vi "8164B CreateLANConnection.vi"(8 "error in":errorcluster, 11 "IP address":string="169.254.2.31") -> (0 "error out":errorcluster, 3 "KeySight 8164B control out":T1)   [LabVIEW 2018, in "KeySight 8164B LAN InstrLib.lvlib"]
uses:
  KeySight 8164B LAN InstrLib.lvlib
  typedefs/KeySight 8164B control.ctl
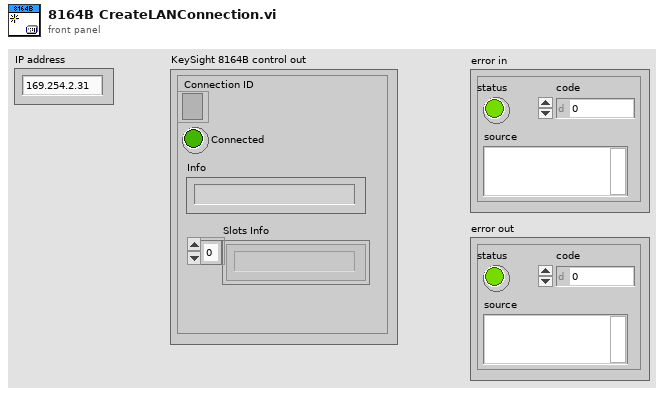
[diagram p1: front panel]
types:
  T1 = typedef "KeySight 8164B LAN InstrLib.lvlib/KeySight 8164B control.ctl" = cluster{"Connection ID":refnum<k5>, "Connected":bool, "Info":string, "Slots Info":string[]}
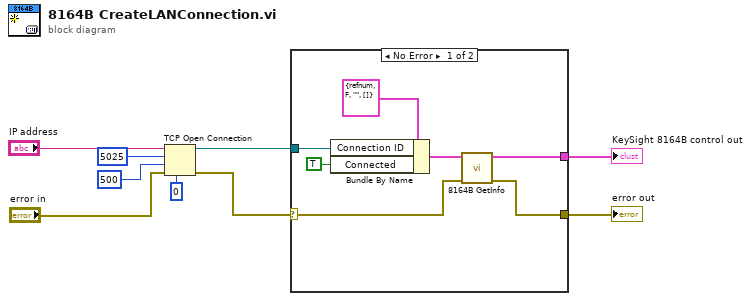
[diagram p0: block diagram]
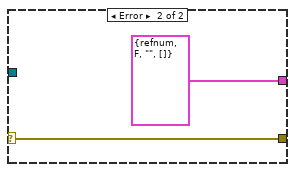
[diagram p2: hidden frame]
diagram:
  n1 = TCP Open Connection(address="IP address", remote port or service name=u16 5025, timeout ms (60000)=500, local port=u16 0 ("local port (0)"), error in (no error)="error in") -> (connection ID=w3:refnum<k5>, error out=w4:errorcluster)
  n2 = case shown="No Error" w4 {
    selector: w4 -> [w11 w17]
    tunnel: w3 -> [w15 _]
    tunnel: [w12 T1 {"Connection ID"=refnum, "Connected"=FALSE, "Info"="", "Slots Info"=[]} ("KeySight 8164B control out")] -> w2
    tunnel: [w10 w17] -> w1
    frame No Error {
      n3 = Bundle By Name(cluster=T1 {"Connection ID"=refnum, "Connected"=FALSE, "Info"="", "Slots Info"=[]} ("KeySight 8164B control out"), "Connection ID"=w15, "Connected"=TRUE) -> (w13:T1)
      n4 = call "8164B GetInfo.vi"("error in"=w11, "KeySight 8164B control in"=w13) -> ("error out"=w10:errorcluster, "KeySight 8164B control out"=w12:T1)  [unwired: 8 in]
    }
    frame Error {
    }
  }
  "KeySight 8164B control out" <- w2
  "error out" <- w1
